vi "Measure Single Point With Compliance.vi"(8 "error in":errorcluster, 11 "niDMM in":refnum<class "niDMM.lvclass">) -> (0 "error out":errorcluster, 1 "Out_Of_Range":bool, 2 "Measured_Value":dbl, 3 "niDMM out":refnum<class "niDMM.lvclass">)   [LabVIEW 2021, in "niDMM.lvclass"]
doc: "Measures the voltage with compliance."
uses:
  niDMM.lvclass
  niDMM.lvclass/niDMM.ctl
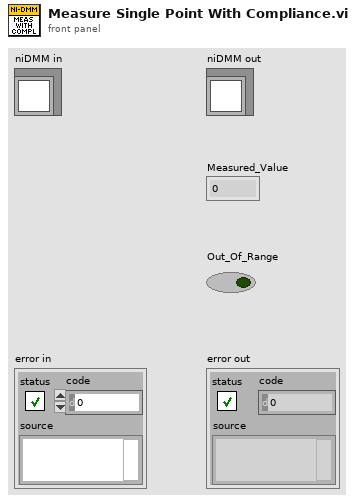
[diagram p1: front panel]
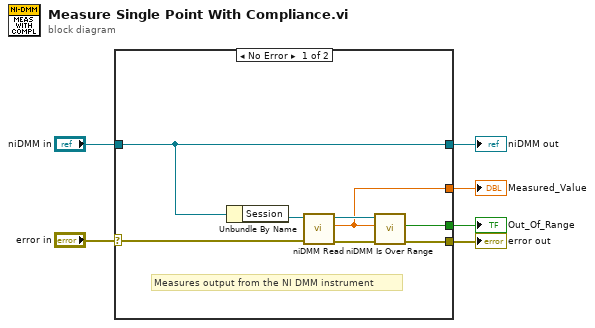
[diagram p0: block diagram]
diagram:
  n1 = case shown="No Error" "error in" {
    selector: "error in" -> [w11 w16]
    tunnel: [w10 w16] -> w5
    tunnel: "niDMM in" -> [w9 w15]
    tunnel: [w9 w15] -> w3
    tunnel: [w8 _] -> w2
    tunnel: [w7 _] -> w1
    frame No Error {
      # "Measures output from the NI DMM instrument"
      n2 = Unbundle By Name(w9) -> ("Session"=w14:refnum<k15>)
      n3 = call <instrlib>:"niDMM Read.vi"("error in (no error)"=w11, "instrument handle"=w14) -> ("error out"=w12:errorcluster, "Measurement"=w7:dbl, "instrument handle out"=w13:refnum<k15>)  [unwired: 7 in]
      n4 = call <instrlib>:"niDMM Is Over Range.vi"("error in (no error)"=w12, "Measurement"=w7, "instrument handle"=w13) -> ("error out"=w10:errorcluster, "Over Range?"=w8:bool)  [unwired: 6 in, 1 out]
    }
    frame Error {
    }
  }
  "error out" <- w5
  "niDMM out" <- w3
  "Measured_Value" <- w1
  "Out_Of_Range" <- w2
